vi "My droplet finder.vi"() -> ()   [LabVIEW 2021]
uses:
  <vilib>/vision/NI_Vision_Development_Module.lvlib
panel:
  out "Analysed Image":T1(plugin-control)
  out "error out":errorcluster
  out "Number of Objects":i32
  out "Objects":T2(array[cluster]) {"Aspect Ratio" format="%.2f"; "Orientation" format="%.2f"; "Area" format="%.2f"; "Object Center"."Y" format="%.2f"; "Object Center"."X" format="%.2f"}
  in  "Settings":T3={"Objects"=0, "Threshold"=1, "Reject Border"=FALSE, "Fill Holes"=TRUE, "Min Object Size"=FALSE, "Min Size"=3, "Max Object Size"=FALSE, "Max Size"=100, "Show Search Area"=FALSE, "Show Center"=TRUE, "Show Bounding Box"=TRUE} {"Objects" items=["Bright Objects", "Dark Objects"]; "Threshold" min=1 max=999999999 step=1; "Max Size" min=1 max=999999999 step=1; "Min Size" min=1 max=999999999 step=1}
  in  "Slide":sgl(slide) scale=0.0..255.0
  in  "stop":bool
  out "Original Image":T1(plugin-control)
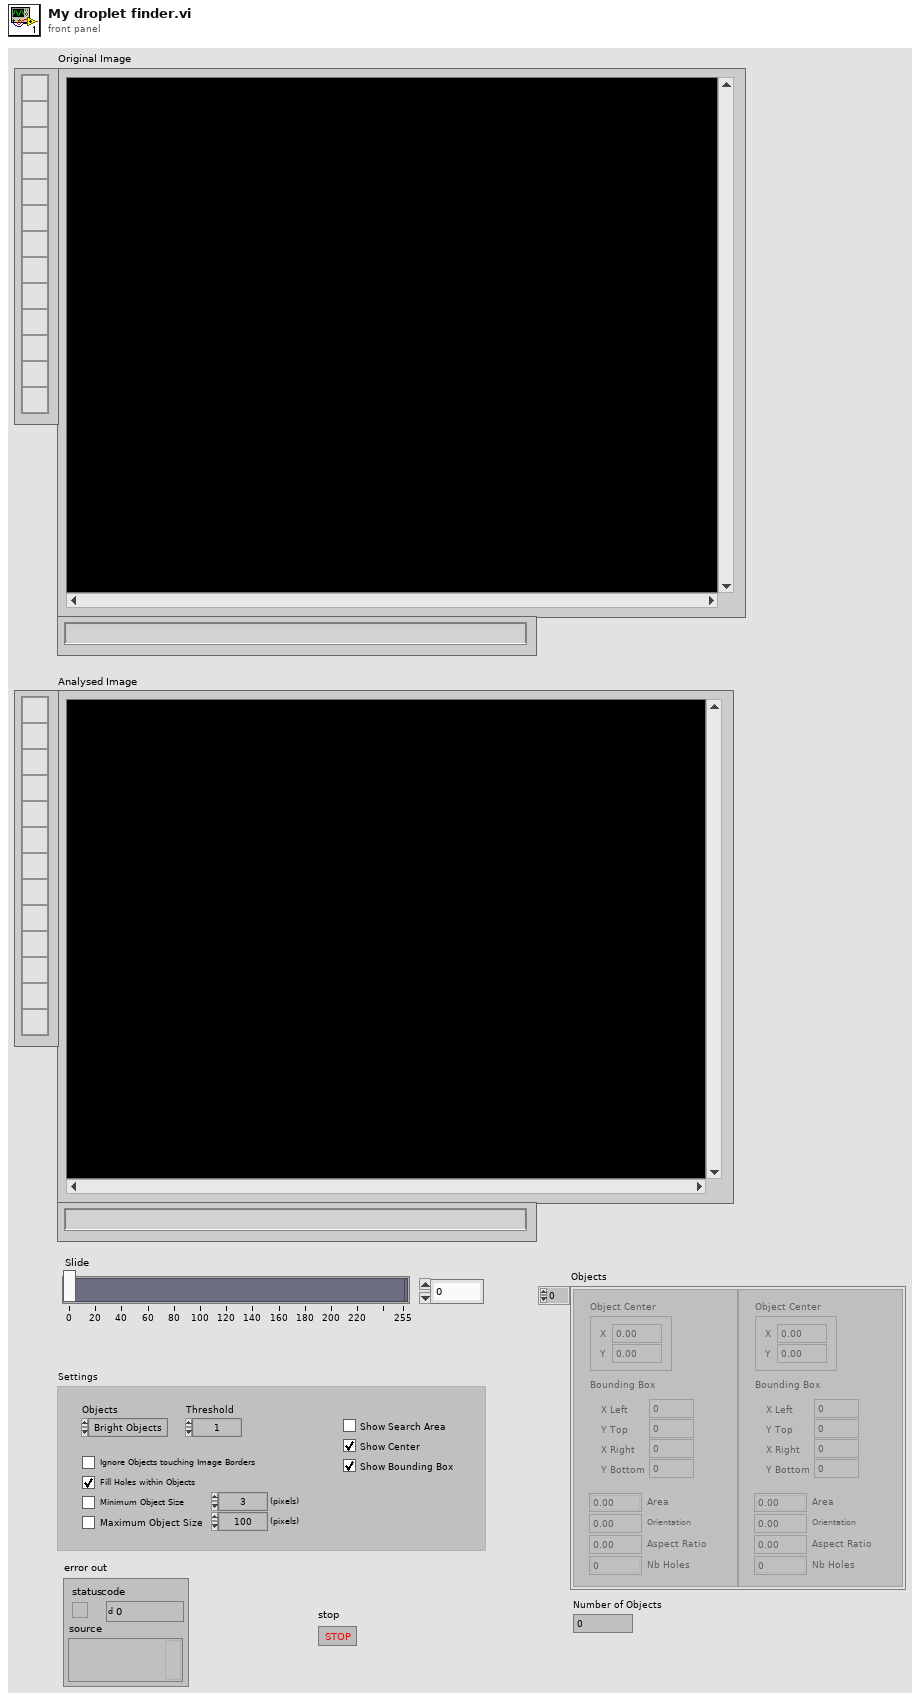
[diagram p1: front panel]
types:
  T1 = typedef "IMAQ Image.ctl" = refnum<image>
  T2 = cluster{"Object Center":cluster{"X":sgl, "Y":sgl}, "Bounding Box":cluster{"X Left":i32, "Y Top":i32, "X Right":i32, "Y Bottom":i32}, "Area":sgl, "Orientation":sgl, "Aspect Ratio":sgl, "Nb Holes":i32}[]
  T3 = cluster{"Objects":u16, "Threshold":i32, "Reject Border":bool, "Fill Holes":bool, "Min Object Size":bool, "Min Size":i32, "Max Object Size":bool, "Max Size":i32, "Show Search Area":bool, "Show Center":bool, "Show Bounding Box":bool}
  T4 = typedef "Image Type" = u32
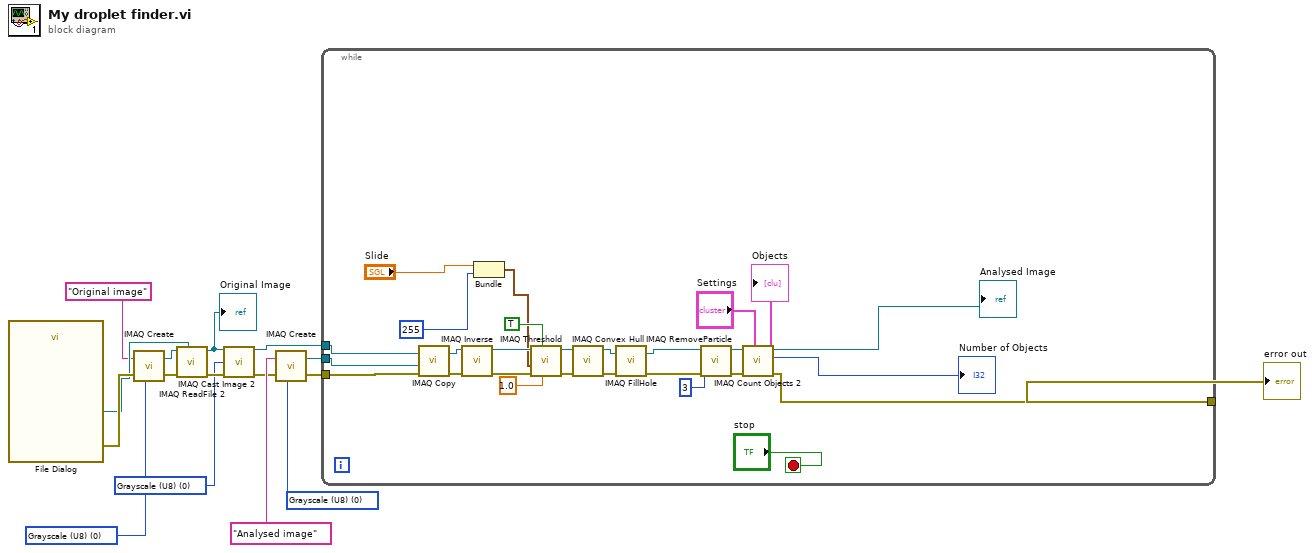
[diagram p0: block diagram]
diagram:
  w2 = T4 0 items=["Grayscale (U8)", "Grayscale (I16)", "Grayscale (SGL)", "Complex (CSG)", "RGB (U32)", "HSL (U32)", "RGB (U64)", "Grayscale (U16)"] ("Image Type")
  w3 = T4 0 items=["Grayscale (U8)", "Grayscale (I16)", "Grayscale (SGL)", "Complex (CSG)", "RGB (U32)", "HSL (U32)", "RGB (U64)", "Grayscale (U16)"] ("Image Type")
  w10 = T4 0 items=["Grayscale (U8)", "Grayscale (I16)", "Grayscale (SGL)", "Complex (CSG)", "RGB (U32)", "HSL (U32)", "RGB (U64)", "Grayscale (U16)"] ("Image Type")
  n1 = call "File Dialog"() -> ("selected path"=w14:path, "error out"=w16:errorcluster)  [unwired: 12 in, 2 out]
  n2 = call "IMAQ Create"("Image Name"="Original image", "Image Type"=w3, "error in (no error)"=w16) -> ("New Image"=w12:T1, "error out"=w15:errorcluster)  [unwired: 2 in]
  n3 = call "IMAQ ReadFile 2"("File Path"=w14, "error in (no error)"=w15, "Image"=w12) -> ("error out"=w11:errorcluster, "Image Out"=w9:T1)  [unwired: 4 in, 3 out]
  "Original Image" <- w9
  n4 = call "IMAQ Cast Image 2"("Image Src"=w9, "Image Type"=w10, "error in (no error)"=w11) -> ("Image Dst Out"=w6:T1, "error out"=w5:errorcluster)  [unwired: 11 in]
  n5 = call "IMAQ Create"("Image Name"="Analysed image", "Image Type"=w2, "error in (no error)"=w5) -> ("New Image"=w7:T1, "error out"=w4:errorcluster)  [unwired: 2 in]
  n6 = while {
    tunnel: w7 -> [w43]
    tunnel: w6 -> [w29]
    tunnel: w4 -> [w42]
    tunnel: [w21] -> w1
    stop <- "stop" stop-if-true
    n7 = call "IMAQ Copy"("error in (no error)"=w42, "Image Dst"=w43, "Image Src"=w29) -> ("error out"=w41:errorcluster, "Image Dst Out"=w34:T1)  [unwired: 3 in]
    n8 = call "IMAQ Inverse"("error in (no error)"=w41, "Image Src"=w34) -> ("error out"=w40:errorcluster, "Image Dst Out"=w33:T1)  [unwired: 8 in]
    n9 = Bundle("Slide"="Slide", 255) -> (w24:cluster{"Slide":sgl, i32})  [unwired: 1 in]
    n10 = call "IMAQ Threshold"("Replace Value"=1.0, "Keep/Replace Value (Replace)"=TRUE, "error in (no error)"=w40, "Range"=w24, "Image Src"=w33) -> ("error out"=w39:errorcluster, "Image Dst Out"=w32:T1)  [unwired: 5 in]
    n11 = call "IMAQ Convex Hull"("error in (no error)"=w39, "Image Src"=w32) -> ("error out"=w38:errorcluster, "Image Dst Out"=w31:T1)  [unwired: 8 in]
    n12 = call "IMAQ FillHole"("error in (no error)"=w38, "Image Src"=w31) -> ("error out"=w17:errorcluster, "Image Dst Out"=w18:T1)  [unwired: 4 in]
    n13 = call "IMAQ RemoveParticle"("error in (no error)"=w17, "Number of Erosion"=3, "Image Src"=w18) -> ("error out"=w37:errorcluster, "Image Dst Out"=w30:T1)  [unwired: 7 in]
    n14 = call "IMAQ Count Objects 2"("Settings"="Settings", "error in (no error)"=w37, "Image"=w30) -> ("error out"=w21:errorcluster, "Number of Objects"=→"Number of Objects":i32, "Image Out"=→"Analysed Image":T1, "Objects"=→"Objects":T2)  [unwired: 4 in, 1 out]
  }
  "error out" <- w1
